vi "Add Channel.vi"(7 "BLRL Type":T1, 8 "error in (no error)":errorcluster, 11 "BluelinesRedlines in":refnum<class "BluelinesRedlines.lvclass">) -> (0 "error out":errorcluster, 3 "BluelinesRedlines out":refnum<class "BluelinesRedlines.lvclass">)   [LabVIEW 2020, in "VolatusGUIElements.lvlib" / "BluelinesRedlines.lvclass"]
uses:
  BluelinesRedlines.lvclass
  VolatusGUI/BluelinesRedlines Source/BLRL Type.ctl
  BluelinesRedlines.lvclass/BluelinesRedlines.ctl
  Volatus/VolatusAPI/VolatusAPI.lvclass
  User BluelinesRedlines/User BluelinesRedlines.lvclass
  C:/dev/lv20CE/relink/lv-volatus/VolatusGUIElements/User BluelinesRedlines/User BluelinesRedlines.lvclass
  C:/dev/lv20CE/relink/lv-volatus/VolatusGUI/BluelinesRedlines Source/BluelinesRedlines Source.lvclass
  VolatusGUI/BluelinesRedlines Source/BluelinesRedlines Source.lvclass
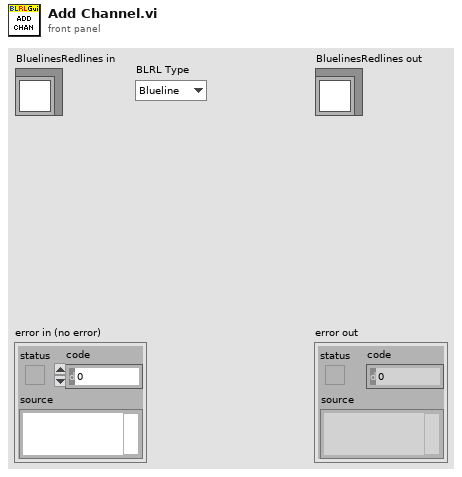
[diagram p1: front panel]
types:
  T1 = typedef "VolatusGUI.lvlib/BluelinesRedlines Source.lvclass/BLRL Type.ctl" = enum16{"Blueline", "Redline"}
  T2 = map{string, refnum<class "BluelinesRedlines Source.lvclass">}
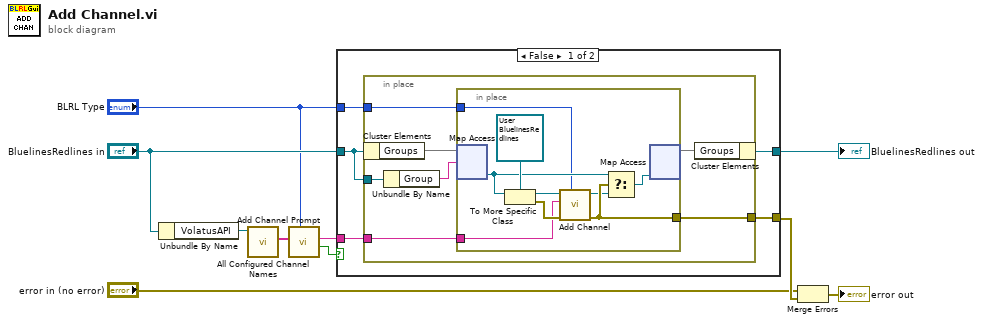
[diagram p0: block diagram]
diagram:
  n1 = Unbundle By Name("BluelinesRedlines in") -> ("VolatusAPI"=w10:refnum<class "VolatusAPI.lvclass">)
  n2 = call "All Configured Channel Names.vi"("VolatusAPI in"=w10) -> ("Channel Names"=w9:string[])  [unwired: 8 in, 2 out]
  n3 = call "Add Channel Prompt.vi"("BLRL Type"="BLRL Type", "Available Channels"=w9) -> ("Cancelled"=w8:bool, "Selected Channel"=w7:string)  [unwired: 8 in]
  n4 = case shown="False" w8 {
    tunnel: w7 -> [w13 _]
    tunnel: "BluelinesRedlines in" -> [w15 w32]
    tunnel: "BLRL Type" -> [w12 _]
    tunnel: [w14 w32] -> w4
    tunnel: [w11 _] -> w3
    frame False {
      n5 = in-place {
        in-place-border: w15 -> [w22]
        in-place-border: w13 -> [w18]
        in-place-border: w12 -> [w17]
        in-place-border: [w16] -> w11
        n6 = in-place-cluster #1(w15) -> ("Groups"=w21:T2)
        n7 = Unbundle By Name(w22) -> ("Group"=w20:string)
        n8 = in-place {
          in-place-border: w18 -> [w25]
          in-place-border: w17 -> [w24]
          in-place-border: [w31] -> w16
          n9 = in-place-map #2(w21, w20) -> (w28:refnum<class "BluelinesRedlines Source.lvclass">)  [unwired: 1 in, 1 out]
          n10 = To More Specific Class(target class=refnum<class "User BluelinesRedlines.lvclass"> refnum ("VolatusGUIElements.lvlib:User BluelinesRedlines.lvclass"), reference=w28) -> (specific class reference=w26:refnum<class "User BluelinesRedlines.lvclass">, error out=w30:errorcluster)  [unwired: 1 in]
          n11 = call "Add Channel.vi"("Type"=w24, "error in (no error)"=w30, "Channel Name"=w25, "User BluelinesRedlines in"=w26) -> ("error out"=w31:errorcluster, "User BluelinesRedlines out"=w23:refnum<class "User BluelinesRedlines.lvclass">)  [unwired: 6 in]
          n12 = Select(t=w28, s=w31, f=w23) -> (s? t:f=w27:refnum<class "BluelinesRedlines Source.lvclass">)
          n13 = in-place-map #2(w27) -> (w19:T2)  [unwired: 1 in, 2 out]
        }
        n14 = in-place-cluster #1("Groups"=w19) -> (w14:refnum<class "BluelinesRedlines.lvclass">)
      }
    }
    frame True {
    }
  }
  "BluelinesRedlines out" <- w4
  n15 = Merge Errors("error in (no error)", w3) -> (→"error out":errorcluster)
